vi "DHT11 Example.vi"() -> ()   [LabVIEW 2009, in "DHT11.lvlib"]
uses:
  DHT11.lvlib
  <vilib>/LabVIEW Interface for Arduino/LabVIEW Interface for Arduino.lvlib
panel:
  in  "stop":bool
  out "Relative Humidity (%)":u8(slide)
  out "Temperature (°C)":u8(slide)
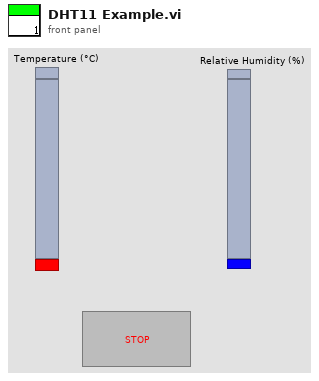
[diagram p1: front panel]
types:
  T1 = typedef "LabVIEW Interface for Arduino.lvlib/Arduino Resource.ctl" = cluster{"VISA resource":refnum<visa-resource-name>, "Board Type":T2, "Connection Type":enum8{"USB / Serial"}, "Bytes Per Packet (15)":u8}
  T2 = typedef "LabVIEW Interface for Arduino.lvlib/Board Type.ctl" = enum16{"Uno", "Dimuelanove w/Atmega 328", "Mega 2560"}
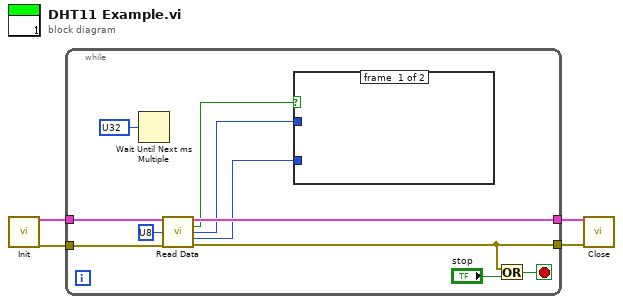
[diagram p0: block diagram]
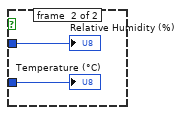
[diagram p2: hidden frame]
diagram:
  n1 = call <vilib>:"Init.vi"() -> ("Arduino Resource"=w4:T1, "error out"=w3:errorcluster)  [unwired: 18 in]
  n2 = while {
    tunnel: w4 -> [w15]
    tunnel: w3 -> [w14]
    tunnel: [w13] -> w2
    tunnel: [w7] -> w1
    stop <- w9 stop-if-true
    n3 = Wait Until Next ms Multiple(millisecond multiple=u32 ?) -> ()  [unwired: 1 out]
    n4 = call "Read Data.vi"("Arduino Resource"=w15, "Pin"=u8 ?, "error in (no error)"=w14) -> ("Arduino Resource"=w13:T1, "Successful?"=w12:bool, "Relative Humidity"=w11:u8, "Temperature (°C)"=w10:u8, "error out"=w7:errorcluster)  [unwired: 8 in]
    n5 = case shown="True" w12 {
      tunnel: w11 -> [_ w16]
      tunnel: w10 -> [_ w17]
      frame #0 {
      }
      frame #1 {
        "Relative Humidity (%)" <- w16
        "Temperature (°C)" <- w17
      }
    }
    n6 = Or(x=w7, y="stop") -> (x .or. y?=w9:bool)
  }
  n7 = call <vilib>:"Close.vi"("Arduino Resource"=w2, "error in"=w1) -> ()  [unwired: 13 in, 1 out]
